vi "ROSPublisher.vi"(2 "Response":T1, 3 "ROS":T2={"topic port"=1236, "Node"="/labview", "topic"="/robot/head/command_head_nod", "type"="std_msgs/Bool", "node port"=7000, "error "={"status"=FALSE, "code"=0, "source"=""}, "Direction"=enum."Publisher", "Update (ms)"=1, "queue size"=1}) -> ()   [LabVIEW 2012]
doc: "Opens new ports for publishers, updates publishers with master, and closes publishers"
uses:
  <userlib>/ROSforLV/ROS/Code/SubVIs/_ROSControl.ctl
  <userlib>/ROSforLV/ROS/Code/SubVIs/_ROSDirection.ctl
  <userlib>/ROSforLV/ROS/Code/_ROSDefinition.vi
panel:
  out "ports":i32[](array[numeric])
  out "Queue log":string
  out "Watchdog":i32
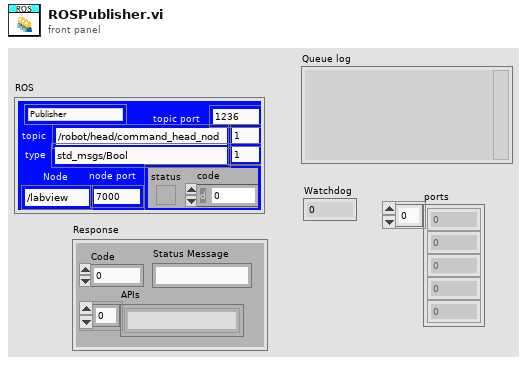
[diagram p1: front panel]
types:
  T1 = cluster{"Code":i32, "Status Message":string, "APIs":string[]}
  T2 = typedef "_ROSControl.ctl" = cluster{"topic port":u16, "Node":string, "topic":string, "type":string, "node port":u16, "error ":errorcluster, "Direction":T3, "Update (ms)":u16, "queue size":u16}
  T3 = typedef "_ROSDirection.ctl" = enum16{"Node", "Publisher", "Subscriber", "Service Client"}
  T4 = enum16{"Reset Log", "Add Client", "Remove Client", "Add Task"}
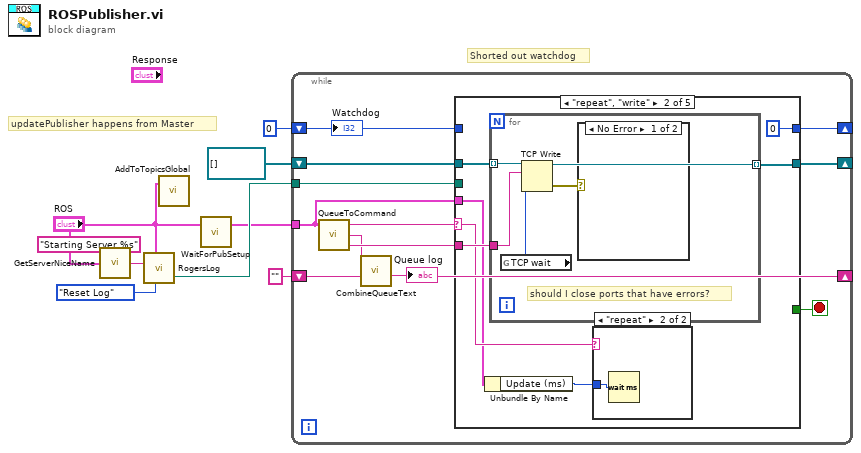
[diagram p0: block diagram]
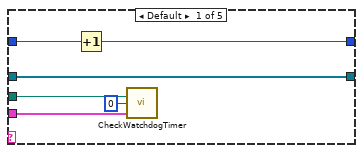
[diagram p2: hidden frame]
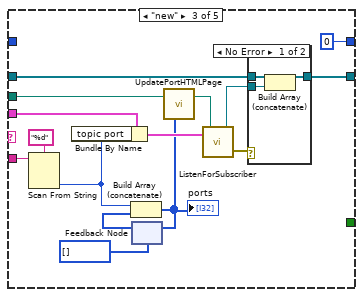
[diagram p5: hidden frame]
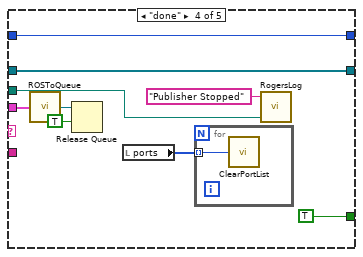
[diagram p7: hidden frame]
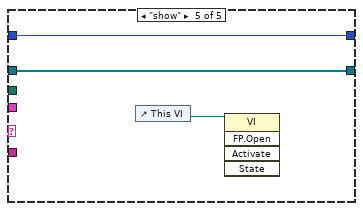
[diagram p8: hidden frame]
diagram:
  # "Shorted out watchdog"
  # "updatePublisher happens from Master"
  n1 = call <userlib>:"GetServerNiceName.vi"("ROS"="ROS", "Text to add"="Starting Server %s") -> ("String"=w8:string)
  n2 = call <userlib>:"RogersLog.vi"("Text to add"=w8, "ROS"="ROS", "Task"=T4."Reset Log") -> ("LogPath out"=w5:path)  [unwired: 2 in, 1 out]
  n3 = call <userlib>:"AddToTopicsGlobal.vi"("ROS in"="ROS") -> ()  [unwired: 3 in]
  n4 = call <userlib>:"WaitForPubSetup.vi"("ROS in"="ROS") -> ("ROS out"=w3:T2)  [unwired: 2 in]
  n5 = while {
    tunnel: w3 -> [w14]
    tunnel: w5 -> [w17]
    shift-right: [w15] -> _
    shift-left: 0 ("timeout ms (wait forever: -1)") -> [w16]
    shift-right: [w13] -> _
    shift-left: refnum<k5>[] [] -> [w20]
    shift-right: [w10] -> _
    shift-left: "" ("New List") -> [w12]
    stop <- w18 stop-if-true
    n6 = call <userlib>:"QueueToCommand.vi"("ROS"=w14) -> ("data"=w19:string, "Queue log"=w11:string, "Command"=w21:string)  [unwired: 2 in]
    n7 = call <userlib>:"CombineQueueText.vi"("Queue in"=w12, "Old List"=w11) -> ("New List"=w10:string)  [unwired: 1 in]
    "Queue log" <- w10
    n8 = case shown="\"repeat\", \"write\"" w21 {
      selector: w21 -> [_ w30 _ _ _]
      tunnel: w20 -> [w26 w32 w52 w64 w70]
      tunnel: w19 -> [_ w34 w54 _ _]
      tunnel: [_ _ _ TRUE _] -> w18
      tunnel: w17 -> [w24 _ w42 w67 _]
      tunnel: w16 -> [w27 _ _ w65 w71]
      tunnel: [w25 0 ("timeout ms (wait forever: -1)") 0 ("timeout ms (wait forever: -1)") w65 w71] -> w15
      tunnel: w14 -> [w23 w28 w44 w60 _]
      tunnel: [w26 w31 w50 w64 w70] -> w13
      frame Default {
        n9 = Increment(x=w27) -> (x+1=w25:i32)
        n10 = call <userlib>:"CheckWatchdogTimer.vi"("ROS"=w23, "itteration"=0, "LogPath in"=w24) -> ()  [unwired: 3 in]
      }
      frame "repeat", "write" {
        n11 = Unbundle By Name(w28) -> ("Update (ms)"=w29:u16)
        n12 = for {
          tunnel: w32 -> [w40] mode=indexing
          tunnel: w34 -> [w39]
          tunnel: [w38] -> w31 mode=indexing
          # "should I close ports that have errors?"
          n13 = global read "_ROSDefinition.vi" "TCP wait"() -> (w37:i32)
          n14 = TCP Write(connection ID=w40, data in=w39, 9:w37) -> (connection ID out=w38:refnum<k5>, error out=w36:errorcluster)  [unwired: 1 in, 1 out]
          n15 = case shown="No Error" w36 {
            frame No Error {
            }
            frame Error {
            }
          }
        }
        n16 = case shown="\"repeat\"" w30 {
          tunnel: w29 -> [_ w35]
          frame Default {
          }
          frame "repeat" {
            n17 = Wait (ms)(milliseconds to wait=w35) -> ()  [unwired: 1 out]
          }
        }
      }
      frame "new" {
        n18 = Scan From String(format string="%d", input string=w54) -> (output 1=w48:i32)  [unwired: 3 in, 3 out]
        n19 = Bundle By Name(cluster=w44, "topic port"=w48) -> (w46:T2)
        n20 = feedback #1(i32[] []) -> (w47:i32[])
        n21 = Build Array (concatenate)(w48, w47) -> (w41:i32[])
        "ports" <- w41
        n22 = feedback-in #1(w41) -> ()
        n23 = call <userlib>:"UpdatePortHTMLPage.vi"("Array"=w41, "LogPath in"=w42) -> ("LogPath out"=w43:path)  [unwired: 1 in]
        n24 = call <userlib>:"ListenForSubscriber.vi"("LogPath in"=w43, "ROS"=w46) -> ("heard?"=w49:errorcluster, "server"=w51:refnum<k5>)
        n25 = case shown="No Error" w49 {
          tunnel: w52 -> [w58 w59]
          tunnel: w51 -> [w57 _]
          tunnel: [w56 w59] -> w50
          frame No Error {
            n26 = Build Array (concatenate)(w58, w57) -> (w56:refnum<k5>[])
          }
          frame Error {
          }
        }
      }
      frame "done" {
        n27 = call <userlib>:"ROSToQueue.vi"("ROS"=w60) -> ("queue"=w62:refnum<queue>)  [unwired: 3 in, 1 out]
        n28 = Release Queue(queue=w62, force destroy? (F)=TRUE) -> ()  [unwired: 1 in, 3 out]
        n29 = local read "ports"() -> (w63:i32[])
        n30 = for {
          tunnel: w63 -> [w69] mode=indexing
          n31 = call <userlib>:"ClearPortList.vi"("topic port"=w69) -> ()  [unwired: 1 in]
        }
        n32 = call <userlib>:"RogersLog.vi"("Text to add"="Publisher Stopped", "LogPath in"=w67) -> ()  [unwired: 3 in, 2 out]
      }
      frame "show" {
        n33 = control-ref of="This VI"() -> (w72:refnum<vi>)
        n34 = invoke class="VI" method="FP.Open"(reference=w72) -> ()  [unwired: 4 in, 5 out]
      }
    }
    "Watchdog" <- w16
  }
